vi "ILS_FTS.vi"() -> ()   [LabVIEW 2010]
uses:
  <vilib>/Analysis/1siggen.llb/Ramp Pattern by Delta.vi
  <vilib>/Analysis/NI_AALBase.lvlib
panel:
  in  "plotextent":dbl=2.0
  out "Total":T1(graph)
  out "Align":T1(graph)
  out "Aperture":T1(graph)
  out "OPD":T1(graph)
  in  "modulation_loss":dbl=0.025
  in  "vEnd":dbl=6165.0
  in  "vStart":dbl=5987.0
  in  "FOV":dbl=0.00296
  in  "OPD":dbl=1.8
  in  "common_grid resolution":dbl=0.01
  in  "ilsextent":dbl=50.0
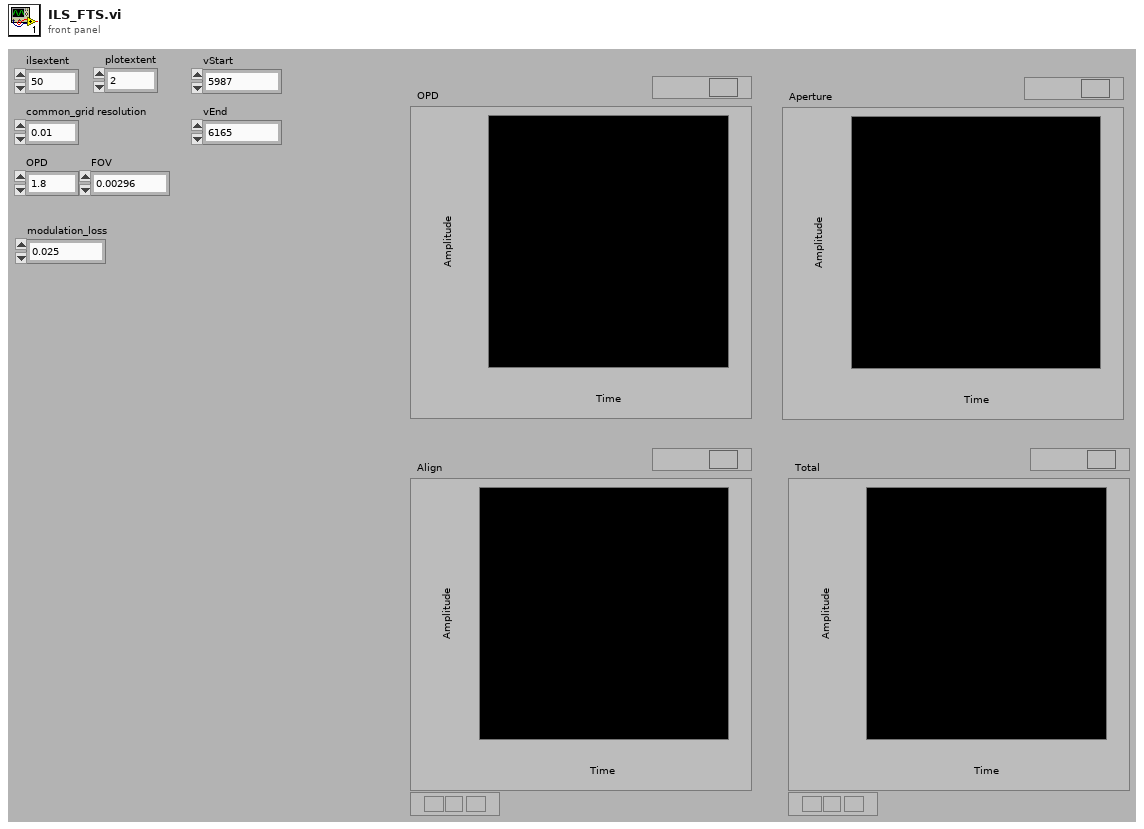
[diagram p1: front panel]
types:
  T1 = cluster{"Ramp Pattern":dbl[], "Sinc Pattern":dbl[]}
  T2 = cluster{"Ramp Pattern":dbl[], "Pulse Pattern":dbl[]}
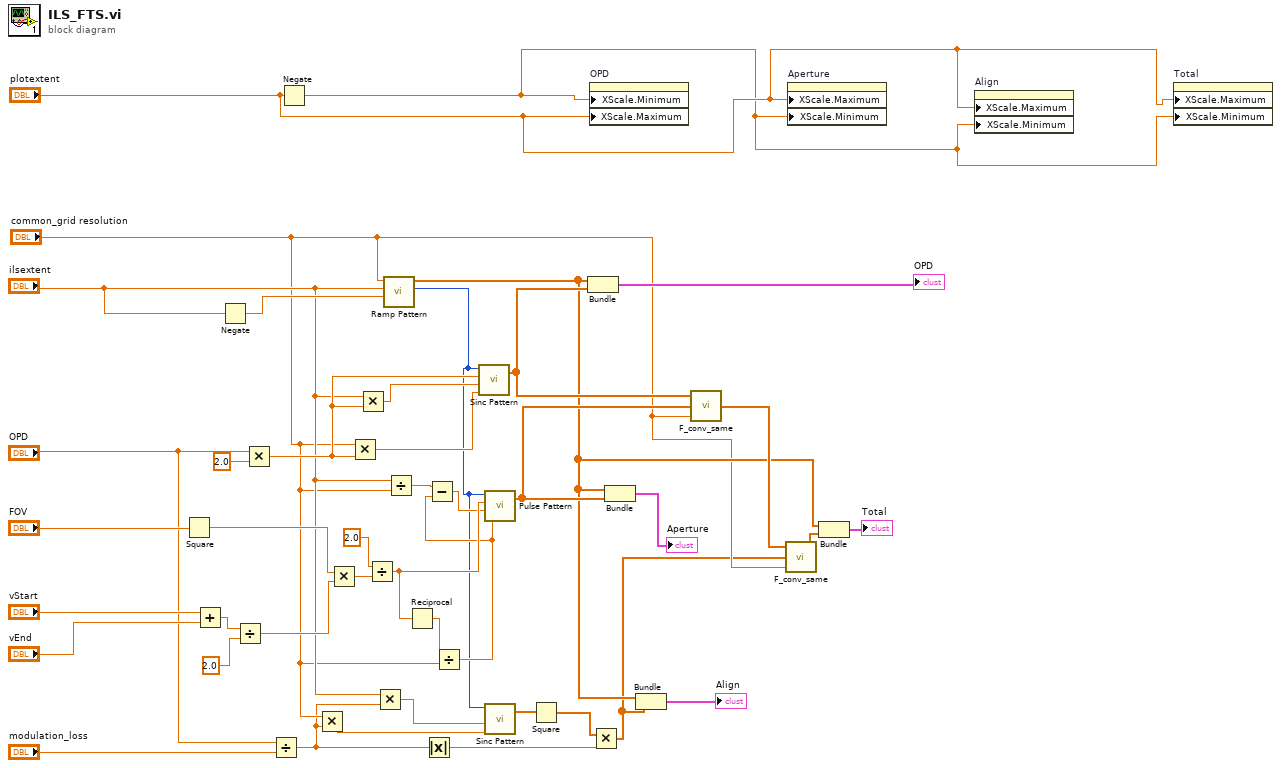
[diagram p0: block diagram]
diagram:
  n1 = Square(x="FOV") -> (x^2=w32:dbl)
  n2 = Add(x="vStart", y="vEnd") -> (x+y=w34:dbl)
  n3 = Negate(x="ilsextent") -> (-x=w42:dbl)
  n4 = Divide(x=w34, y=2.0) -> (x/y=w31:dbl)
  n5 = Multiply(x="OPD", y=2.0) -> (x*y=w38:dbl)
  n6 = Divide(x="OPD", y="modulation_loss") -> (x/y=w4:dbl)
  n7 = Negate(x="plotextent") -> (-x=w6:dbl)
  n8 = Multiply(x="common_grid resolution", y=w4) -> (x*y=w20:dbl)
  n9 = Multiply(x=w32, y=w31) -> (x*y=w30:dbl)
  n10 = Multiply(x="common_grid resolution", y=w38) -> (x*y=w40:dbl)
  n11 = Multiply(x="ilsextent", y=w38) -> (x*y=w39:dbl)
  n12 = Divide(x=2.0 ("y"), y=w30) -> (x/y=w28:dbl)
  n13 = Multiply(x="ilsextent", y=w4) -> (x*y=w18:dbl)
  n14 = call-poly <vilib>:"Ramp Pattern.vi"("start"=w42, "end"="ilsextent", "delta"="common_grid resolution") -> ("samples"=w23:i32, "Ramp Pattern"=w8:dbl[])  [unwired: 6 in, 1 out]
  n15 = Divide(x="ilsextent", y="common_grid resolution") -> (x/y=w26:dbl)
  n16 = Reciprocal(x=w28) -> (1/x=w27:dbl)
  n17 = Absolute Value(x=w4) -> (abs(x)=w3:dbl)
  n18 = Divide(x=w27, y="common_grid resolution") -> (x/y=w25:dbl)
  n19 = Subtract(x=w26, y=w25) -> (x-y=w24:dbl)
  n20 = call <vilib>:"Sinc Pattern.vi"("delta t"=w40, "delay"=w39, "amplitude"=w38, "samples"=w23) -> ("Sinc Pattern"=w16:dbl[])  [unwired: 1 out]
  n21 = call <vilib>:"Pulse Pattern.vi"("width"=w25, "delay"=w24, "amplitude"=w28, "samples"=w23) -> ("Pulse Pattern"=w13:dbl[])  [unwired: 1 out]
  n22 = call <vilib>:"Sinc Pattern.vi"("delta t"=w20, "delay"=w18, "samples"=w23) -> ("Sinc Pattern"=w17:dbl[])  [unwired: 1 in, 1 out]
  n23 = Square(x=w17) -> (x^2=w2:dbl[])
  n24 = Bundle("Ramp Pattern"=w8, "Sinc Pattern"=w16) -> (→"OPD":T1)  [unwired: 1 in]
  n25 = property on="OPD" class="XYGraph (strict)"("XScale.Minimum"=w6, "XScale.Maximum"="plotextent") -> ()  [unwired: 2 in, 2 out]
  n26 = Multiply(x=w2, y=w3) -> (x*y=w1:dbl[])
  n27 = Bundle("Ramp Pattern"=w8, "Pulse Pattern"=w13) -> (→"Aperture":T2)  [unwired: 1 in]
  n28 = Bundle("Ramp Pattern"=w8, w1) -> (→"Align":cluster{"Ramp Pattern":dbl[], dbl[]})  [unwired: 1 in]
  n29 = call "F_conv_same.vi"("dt"="common_grid resolution", "Pulse Pattern"=w13, "Sinc Pattern"=w16) -> ("Convolved"=w11:dbl[])
  n30 = call "F_conv_same.vi"("dt"="common_grid resolution", "Pulse Pattern"=w1, "Sinc Pattern"=w11) -> ("Convolved"=w9:dbl[])
  n31 = property on="Aperture" class="XYGraph (strict)"("XScale.Maximum"="plotextent", "XScale.Minimum"=w6) -> ()  [unwired: 2 in, 2 out]
  n32 = Bundle("Ramp Pattern"=w8, "Convolved"=w9) -> (→"Total":cluster{"Ramp Pattern":dbl[], "Convolved":dbl[]})  [unwired: 1 in]
  n33 = property on="Align" class="XYGraph (strict)"("XScale.Maximum"="plotextent", "XScale.Minimum"=w6) -> ()  [unwired: 2 in, 2 out]
  n34 = property on="Total" class="XYGraph (strict)"("XScale.Maximum"="plotextent", "XScale.Minimum"=w6) -> ()  [unwired: 2 in, 2 out]
